vi "BracePLUS_File_Viewer.vi"(11 "Path":path) -> (0 "error out":errorcluster)   [LabVIEW 2018]
uses:
  <vilib>/Math Plots/3D Math Plots/3D Surface/3D Surface XCtrl/3D Surface.xctl
  subVIs/calibration/FGVs/FGV States.ctl
  <vilib>/Utility/file.llb/Write Delimited Spreadsheet (DBL).vi
  <vilib>/Utility/file.llb/Read Delimited Spreadsheet (I64).vi
  <vilib>/Math Plots/3D Math Plots/3D Surface/3D Surface Datatype/Public/Plot Helper (Matrix).vi
  <vilib>/Math Plots/3D Math Plots/3D Surface/3D Surface Datatype/3D Surface Datatype.lvclass
panel:
  in  "Slider":i32(slide) scale=0.0..4881.0
  in  "Tab Control":T1(tab)
  out "3D Surface":refnum<class "3D Plot Datatype.lvclass">[](xcontrol)
  out "Calibrated Output":dbl[][](array[numeric]) format="%.2f"
  in  "dT":u32=40
  out "Data Packet":string
  out "Time":u32=4294745741
  out "Read Count":i32
  out "Lookup Indices":i32[](array[numeric])=[0, 4, 8, 12, 1, 5, 9, 13, 16, 20, 24, 28, 17, 21, 25, 29, 15, 11, 7, 3, 14, 10, 6, 2, 31, 27, 23, 19, 30, 26, 22, 18, 32, 36, 40, 44, 33, 37, 41, 45, 48, 52, 56, 60, 49, 53, 57, 61, 47, 43, 39, 35, 46, 42, 38, 34, 63, 59, 55, 51, 62, 58, 54, 50, 64, 68, 72, 76, 65, 69, 73, 77, 80, 84, 88, 92, 81, 85, 89, 93, 79, 75, 71, 67, 78, 74, 70, 66, 95, 91, 87, 83, 94, 90, 86, 82, 96, 100, 104, 108, 97, 101, 105, 109, 112, 116, 120, 124, 113, 117, 121, 125, 111, 107, 103, 99, 110, 106, 102, 98, 127, 123, 119, 115, 126, 122, 118, 114]
  in  "Calibration File":string="Magboard_Btod_new_calib"
  in  "Packet Size (Bytes)":u32=1024
  in  "Gains":dbl[](array[numeric])=[0.751, 0.751, 1.21]
  in  "Export File (CSV)":path=path "C:/Users/menprc/Documents/GitHub/MagLib/MagBoard_n64_UI/MagBoard_n64_UI_LabVIEW_Client/example_data/M064_008.csv"
  in  "Save?":bool
  in  "Upper Limit":dbl=1.0 format="%#_13g"
  in  "Lower Limit":dbl=-10.0 format="%#_13g"
  out "Filesize (bytes)":i64
  out "No. Packets":dbl
  in  "Tare?":bool
  out "Calibrated Output":dbl[][](array[numeric])
  out "B xyz":dbl[][](array[numeric]) format="%#.0f"
  in  "stop":bool
  # "ESCAPES: File Viewer"
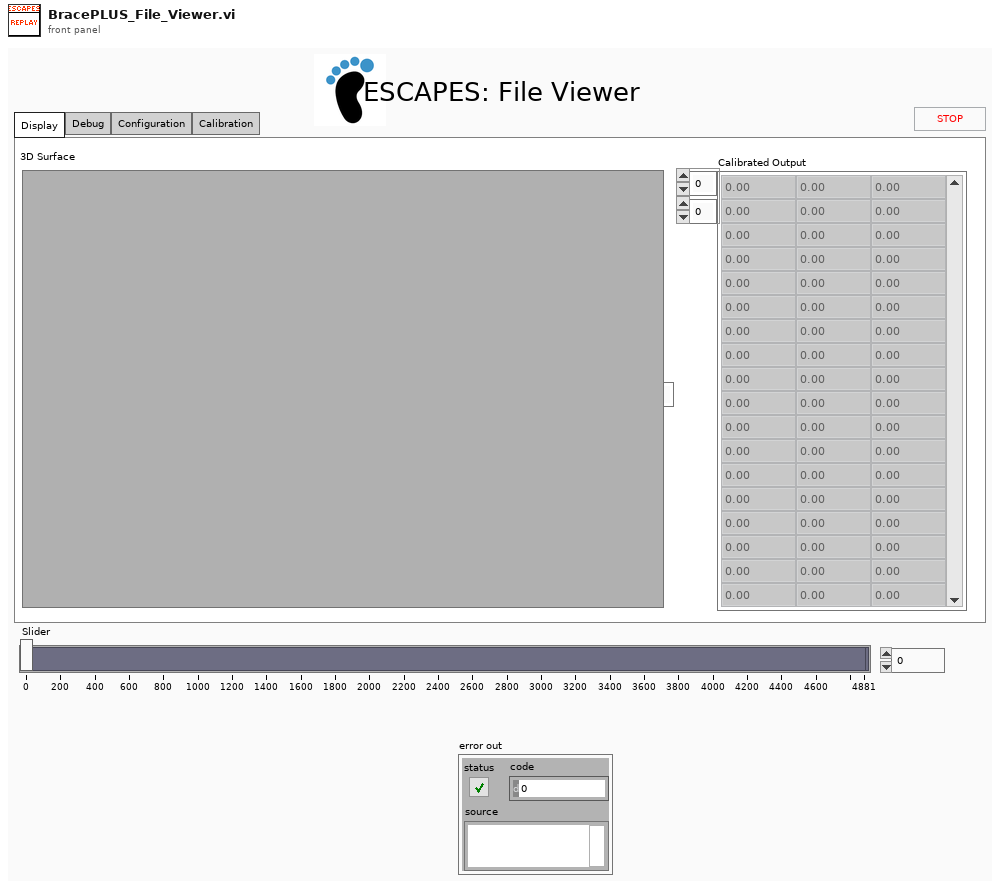
[diagram p1: front panel]
types:
  T1 = enum32{"Display", "Debug", "Configuration", "Calibration"}
  T2 = typedef "FGV States.ctl" = enum16{"Get", "Set", "Reset"}
  T3 = cluster{cluster{dbl[][], "Array":dbl[][]}, cluster{dbl[][], "Array":dbl[][]}, cluster{dbl[][], "Array":dbl[][]}, cluster{dbl[][], "Array":dbl[][]}}
  T4 = cluster{cluster{dbl[][], "Array":dbl[][]}, cluster{dbl[][], "Array":dbl[][]}, cluster{dbl[][], "Array":dbl[][]}, cluster{dbl[][], "Array":dbl[][]}}[]
  T5 = enum16{"big-endian, network order", "native, host order", "little-endian"}
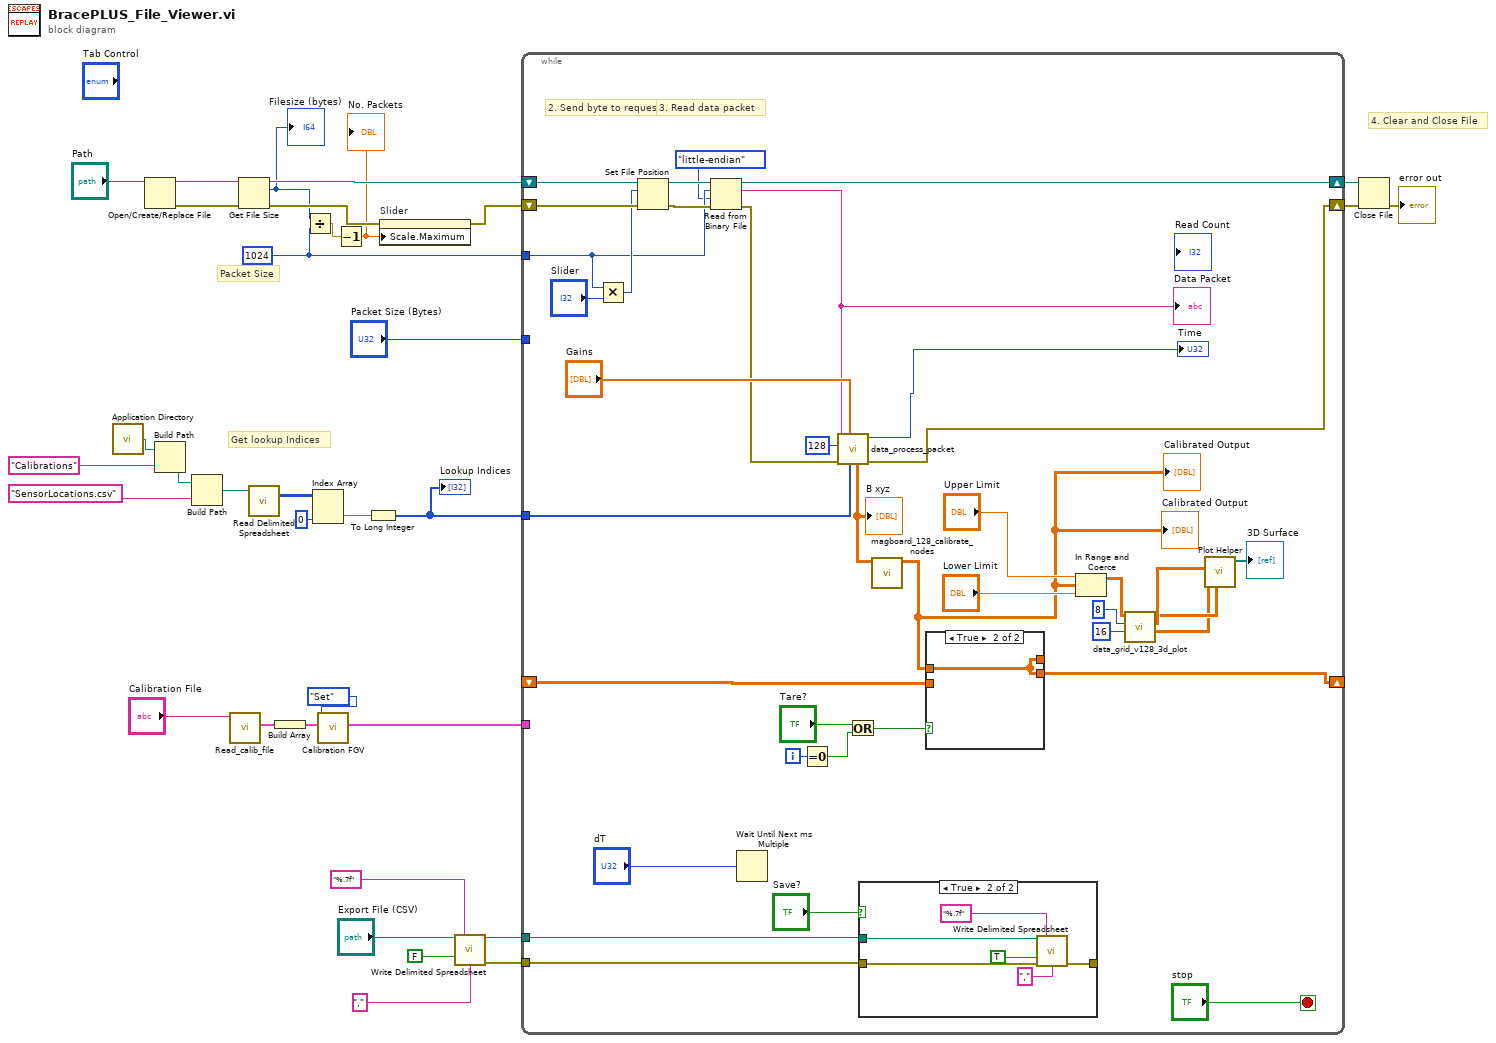
[diagram p0: block diagram]
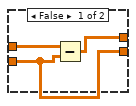
[diagram p2: hidden frame]
diagram:
  w8 = 1024 ("count (1)")
  # "Packet Size"
  # "Get lookup Indices"
  # "4. Clear and Close File"
  n1 = call <vilib>:"Application Directory.vi"() -> ("Application Directory"=w3:path)
  n2 = Open/Create/Replace File(file path (use dialog)="Path") -> (refnum out=w15:refnum<file>, error out=w14:errorcluster)  [unwired: 5 in, 1 out]
  n3 = Build Path(base path=w3, name or relative path="Calibrations" ("string")) -> (appended path=w5:path)
  n4 = Build Path(base path=w5, name or relative path="SensorLocations.csv" ("string")) -> (appended path=w2:path)
  n5 = call "Read_calib_file.vi"("string"="Calibration File") -> ("output cluster"=w23:T3)  [unwired: 6 in, 4 out]
  n6 = Get File Size(file=w15, error in=w14) -> (refnum out=w13:refnum<file>, size (in bytes)=w9:i64, 0:w12:errorcluster)
  "Filesize (bytes)" <- w9
  n7 = call-poly <vilib>:"Read Delimited Spreadsheet.vi"("file path (dialog if empty)"=w2) -> ("all rows"=w26:i64[][])  [unwired: 9 in, 5 out]
  n8 = Build Array(w23) -> (w22:T4)
  n9 = Divide(x=w9, y=w8) -> (x/y=w10:dbl)
  n10 = Index Array(array=w26, index (col)=0 ("disabled index (col)")) -> (element=w24:i64[])  [unwired: 1 in]
  n11 = call "Calibration FGV.vi"("Calib in"=w22, "FGV States"=FGV_States."Set") -> ("Calib in 2"=w20:T4)  [unwired: 9 in]
  n12 = Decrement(x=w10) -> (x-1=w7:dbl)
  "No. Packets" <- w7
  n13 = To Long Integer(number=w24) -> (32bit integer=w33:i32[])
  "Lookup Indices" <- w33
  n14 = property on="Slider" class="Slide (strict)"(error in=w12, "Scale.Maximum"=w7) -> (error out=w11:errorcluster)  [unwired: 1 in, 1 out]
  n15 = call-poly <vilib>:"Write Delimited Spreadsheet.vi"("file path (dialog if empty)"="Export File (CSV)", "format (%.3f)"="%.7f", "append to file? (new file:F)"=FALSE, "delimiter (\\t)"="," ("delimiter (\\t)")) -> ("new file path (Not A Path if cancelled)"=w28:path, "error out"=w27:errorcluster)  [unwired: 10 in]
  n16 = while {
    shift-right: [w55] -> w17
    shift-left: w13 -> [w57]
    tunnel: w33 -> [w69]
    shift-right: [w65] -> w18
    shift-left: w11 -> [w56]
    tunnel: "Packet Size (Bytes)" -> [_]
    tunnel: w28 -> [w64]
    tunnel: w27 -> [w63]
    tunnel: w20 -> [_]
    shift-right: [w58] -> _
    shift-left: _ -> [w59]
    tunnel: w8 -> [w44]
    i -> [w68]
    stop <- "stop" stop-if-true
    # "3. Read data packet"
    # "2. Send byte to request reading"
    n17 = Multiply(x=w44, y="Slider") -> (x*y=w45:i32)
    n18 = Set File Position(offset (in bytes) (0)=w45, refnum=w57) -> (refnum out=w47:refnum<file>)  [unwired: 2 in, 1 out]
    n19 = Read from Binary File(8:w56, 9:T5."little-endian" ("byte order (0:big-endian, network order)"), 10:w44, 11:w47) -> (0:w54:errorcluster, 2:w48:string, 3:w55:refnum<file>)  [unwired: 2 in, 1 out]
    "Data Packet" <- w48
    n20 = Wait Until Next ms Multiple(millisecond multiple="dT") -> ()  [unwired: 1 out]
    n21 = Equal To 0?(x=w68) -> (x = 0?=w50:bool)
    n22 = call "data_process_packet.vi"("Sensor Lookup Indices"=w69, "Gains"="Gains", "error in (no error)"=w54, "No. Sensors"=128 ("No. Nodes"), "Binary Input Data"=w48) -> ("error out"=w65:errorcluster, "Time"=→"Time":u32, "Sensors (uT)"=w61:dbl[][])  [unwired: 2 in, 2 out]
    "B xyz" <- w61
    n23 = Or(x="Tare?", y=w50) -> (x .or. y?=w51:bool)
    n24 = case shown="True" "Save?" {
      tunnel: w64 -> [_ w79]
      tunnel: w63 -> [w76 w78]
      tunnel: [w76 w77] -> _
      frame False {
      }
      frame True {
        n25 = call-poly <vilib>:"Write Delimited Spreadsheet.vi"("file path (dialog if empty)"=w79, "format (%.3f)"="%.7f", "append to file? (new file:F)"=TRUE, "error in (no error)"=w78, "delimiter (\\t)"="," ("delimiter (\\t)")) -> ("error out"=w77:errorcluster)  [unwired: 9 in, 1 out]
      }
    }
    n26 = call "magboard_128_calibrate_nodes.vi"("Sensor Input (mT)"=w61) -> ("Sensor Output - Position (mm)"=w36:dbl[][])  [unwired: 10 in]
    "Calibrated Output" <- w36
    "Calibrated Output" <- w36
    n27 = case shown="True" w51 {
      tunnel: w36 -> [w74 w75]
      tunnel: w59 -> [w73 _]
      tunnel: [w73 w75] -> w58
      tunnel: [w72 w75] -> _
      frame False {
        n28 = Subtract(x=w74, y=w73) -> (x-y=w72:dbl[][])
      }
      frame True {
      }
    }
    n29 = In Range and Coerce(upper limit="Upper Limit", x=w36, lower limit="Lower Limit") -> (coerced(x)=w42:dbl[][])  [unwired: 1 out]
    n30 = call "data_grid_v128_3d_plot.vi"("No. Rows"=16 ("Row Length"), "No. Columns"=8, "Sensor Data"=w42) -> ("Y (GRID)"=w37:dbl[][], "X (GRID)"=w39:dbl[][], "Z (GRID)"=w38:dbl[][])  [unwired: 6 in]
    n31 = call-poly <vilib>:"Plot Helper.vi"("z matrix"=w38, "y matrix"=w37, "x matrix"=w39) -> ("3D Plot lvclass Array out"=→"3D Surface":refnum<class "3D Plot Datatype.lvclass">[])  [unwired: 3 in, 5 out]
  }
  n32 = Close File(refnum=w17, error in=w18) -> (error out=→"error out":errorcluster)  [unwired: 1 out]
